vi "channel_vrs_time_cluster.vi"(2 "?":T1=enum."VCC", 3 "Clear Graph?":bool, 4 "Time":dbl, 5 "Input data":dbl[][](array[numeric])) -> (0 "Cluster":cluster{dbl[], dbl[]}, 1 "rms value":dbl format="%0.2f")   [LabVIEW 2016]
uses:
  INPUTS.ctl
  <vilib>/Analysis/5stat.llb/RMS (DBL).vi
  <vilib>/Analysis/NI_AALPro.lvlib
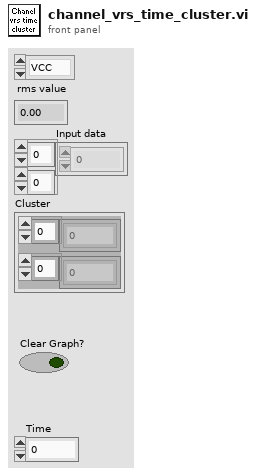
[diagram p1: front panel]
types:
  T1 = typedef "INPUTS.ctl" = enum16{"I_CELL", "I_LOAD", "I_PV", "V_BUS", "V_CELL", "VCC"}
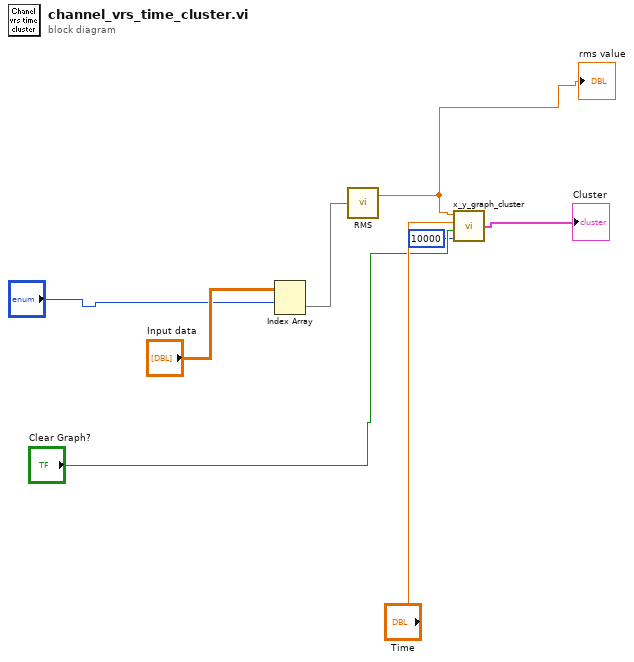
[diagram p0: block diagram]
diagram:
  n1 = Index Array(array="Input data", index (row)="?") -> (element=w8:dbl[])  [unwired: 1 in]
  n2 = call-poly <vilib>:"RMS.vi"("X"=w8) -> ("rms value"=w1:dbl)  [unwired: 1 out]
  "rms value" <- w1
  n3 = call "x_y_graph_cluster.vi"("Chart History (10,000)"=10000, "Clear Graph?"="Clear Graph?", "X"="Time", "Y"=w1) -> ("Cluster"=→"Cluster":cluster{dbl[], dbl[]})
